vi "InventoryTree-DeleteSingleTag.vi"(7 "Work Order":string, 8 "error in (no error)":errorcluster, 11 "ERP-Inventory in":refnum<class "ERP-Inventory.lvclass">) -> (0 "error out":errorcluster, 3 "ERP-Inventory out":refnum<class "ERP-Inventory.lvclass">)   [LabVIEW 2013, in "ERP-Inventory.lvclass"]
uses:
  ERP-Inventory.lvclass
  ERP-Inventory.lvclass/ERP-Inventory.ctl
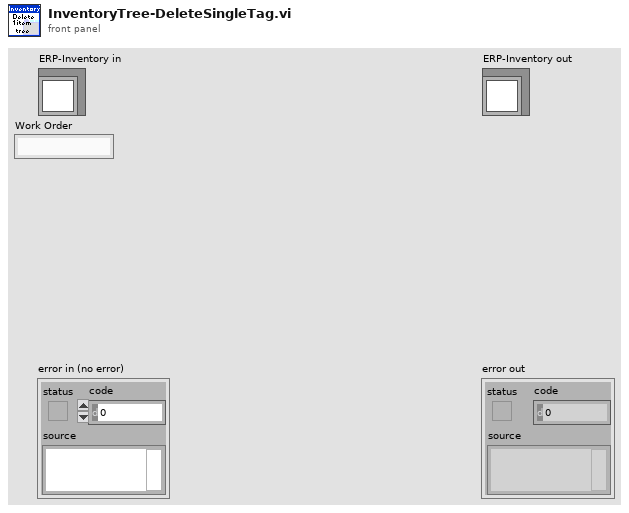
[diagram p1: front panel]
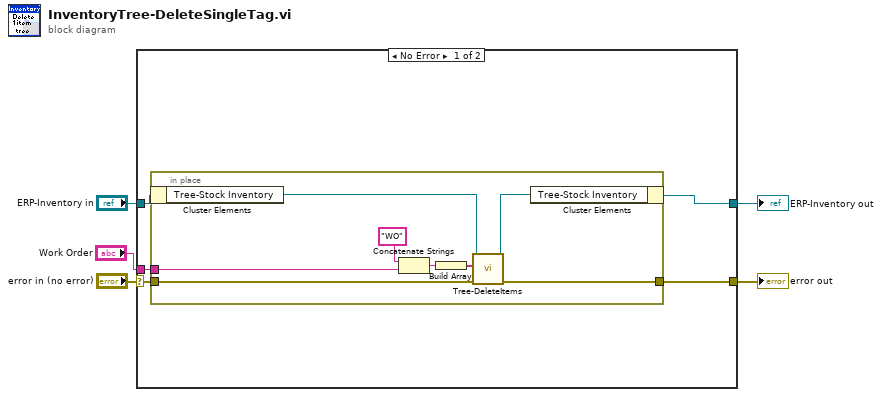
[diagram p0: block diagram]
diagram:
  n1 = case shown="No Error" "error in (no error)" {
    selector: "error in (no error)" -> [w10 w20]
    tunnel: [w9 w20] -> w4
    tunnel: [w7 w19] -> w2
    tunnel: "ERP-Inventory in" -> [w8 w19]
    tunnel: "Work Order" -> [w6 _]
    frame No Error {
      n2 = in-place {
        in-place-border: w10 -> [w13]
        in-place-border: [w12] -> w9
        in-place-border: w6 -> [w11]
        n3 = in-place-cluster #1(w8) -> ("Tree-Stock Inventory"=w17:refnum<vi>)
        n4 = Concatenate Strings("WO", w11) -> (w15:string)
        n5 = Build Array(w15) -> (w14:string[])
        n6 = call "Tree-DeleteItems.vi"("error In"=w13, "All Tags"=w14, "Tree In"=w17) -> ("error out"=w12:errorcluster, "Tree out"=w18:refnum<vi>)  [unwired: 7 in]
        n7 = in-place-cluster #1("Tree-Stock Inventory"=w18) -> (w7:refnum<class "ERP-Inventory.lvclass">)
      }
    }
    frame Error {
    }
  }
  "error out" <- w4
  "ERP-Inventory out" <- w2
